vi "DC-DC_SC.vi"() -> ()   [LabVIEW 2025]
uses:
  controls/DC-DC-SC-2-enum.ctl
  controls/DC-DC-SC-2-cluster.ctl
  <vilib>/Utility/file.llb/Write Delimited Spreadsheet (string).vi
  <instrlib>/BK Precision 9200 Series/BK Precision 9200 Series.lvlib
panel:
  out "Time":u32
  in  "Current :":dbl
  in  "Voltage :":dbl
  in  "START":bool
  in  "BK_COM :":refnum<visa-resource-name>
  out "error out":errorcluster
  in  "error in (no error)":errorcluster
  in  "DATA":i32(listbox)
  in  "Exit":bool
  in  "Connect":bool
  # "DC-DC-Shorts"
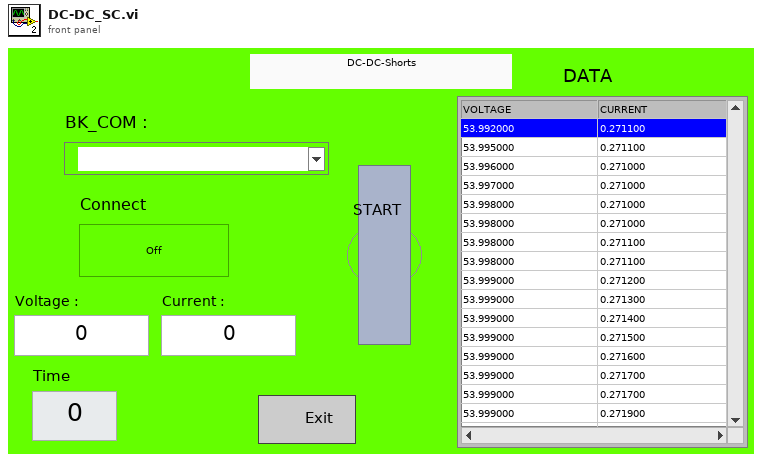
[diagram p1: front panel]
types:
  T1 = typedef "DC-DC-SC-2-cluster.ctl" = cluster{"File":path, "BK COM":refnum<visa-resource-name>, "Data":string[], "Stop":bool, "Start":bool, "Parameters":dbl[], "Seconds":u32}
  T2 = typedef "DC-DC-SC-2-enum.ctl" = enum16{"Init", "Poll", "Connect", "Set", "Start", "Read", "Stop", "Log", "Error", "Exit"}
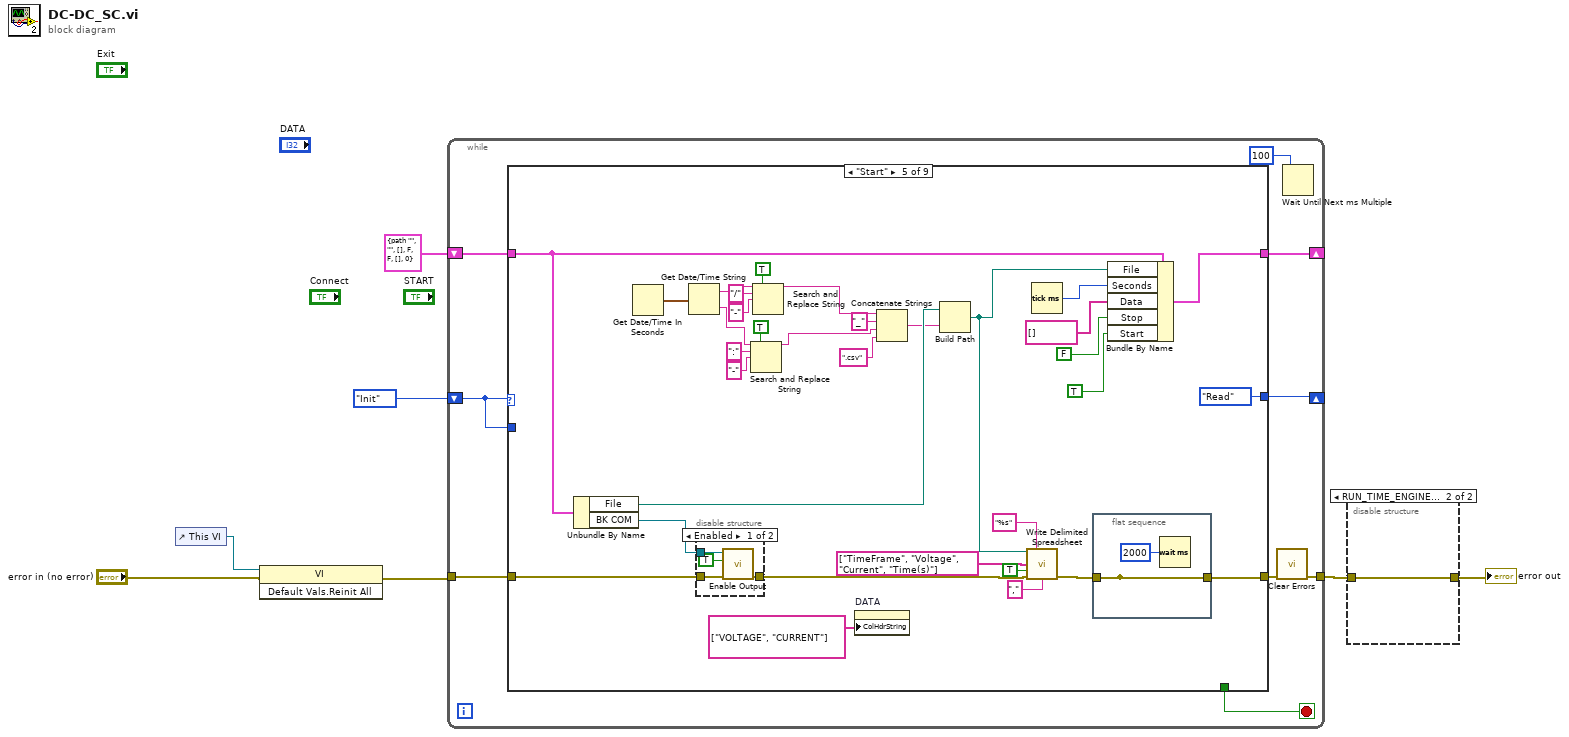
[diagram p0: block diagram]
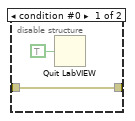
[diagram p2: hidden frame]
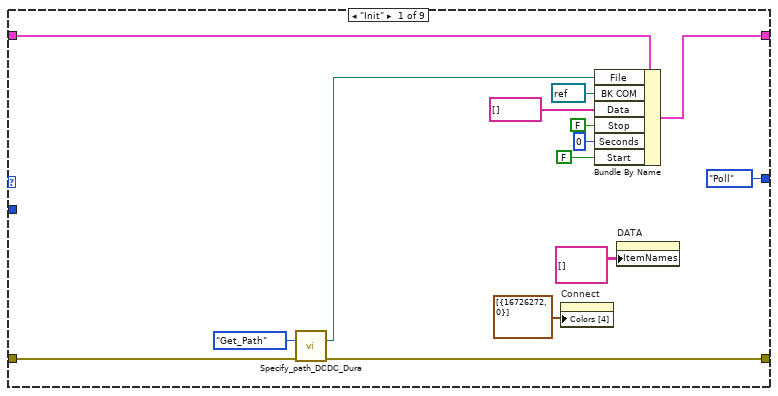
[diagram p3: hidden frame]
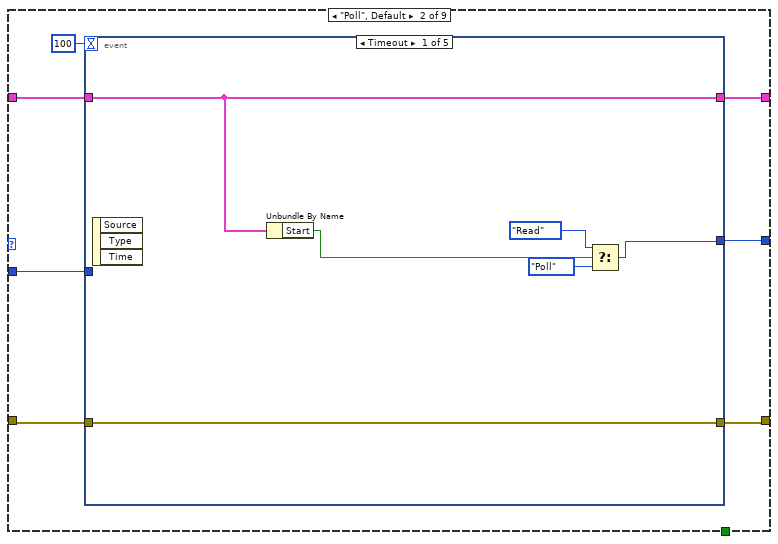
[diagram p4: hidden frame]
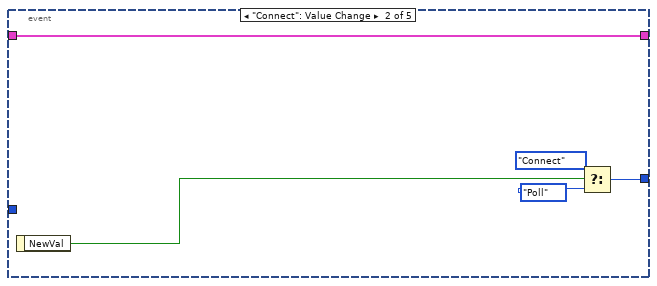
[diagram p5: hidden frame]
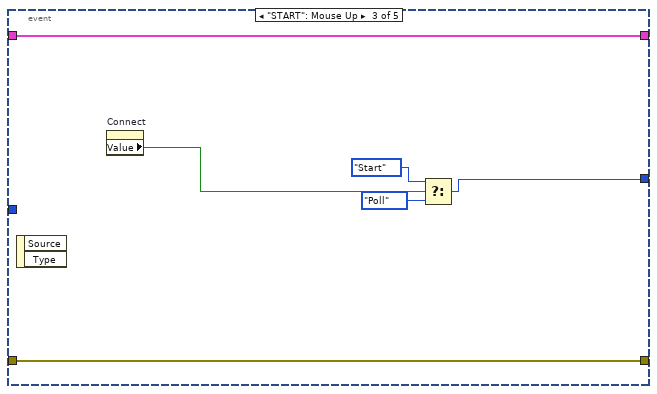
[diagram p6: hidden frame]
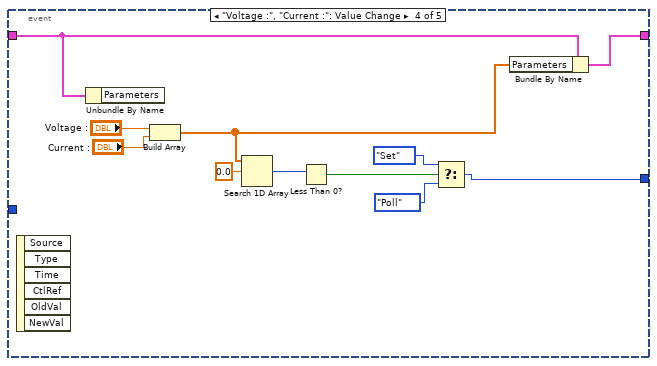
[diagram p7: hidden frame]
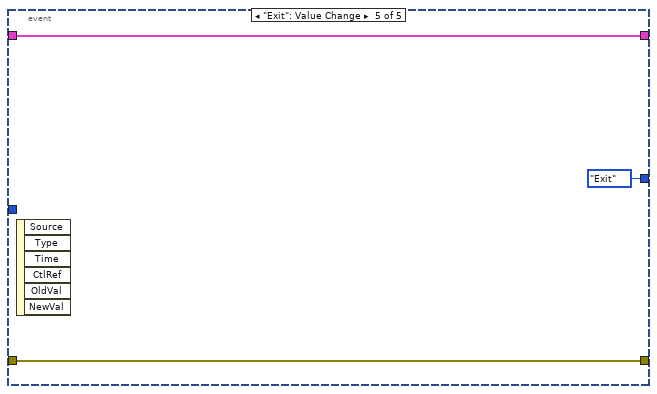
[diagram p8: hidden frame]
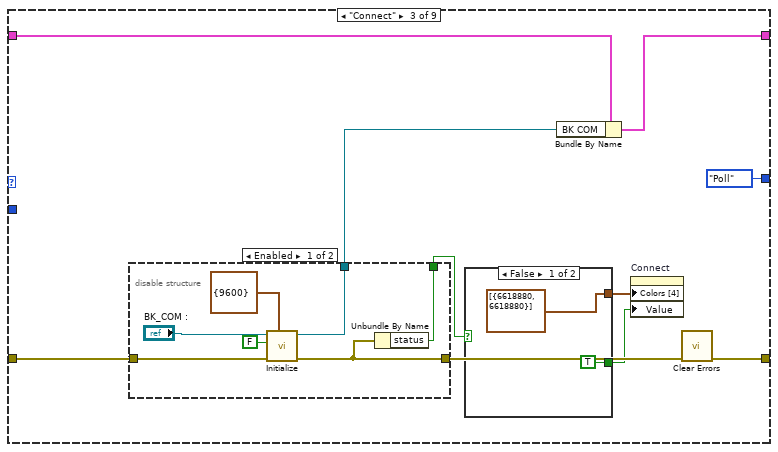
[diagram p9: hidden frame]
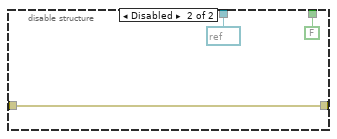
[diagram p10: hidden frame]
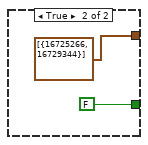
[diagram p11: hidden frame]
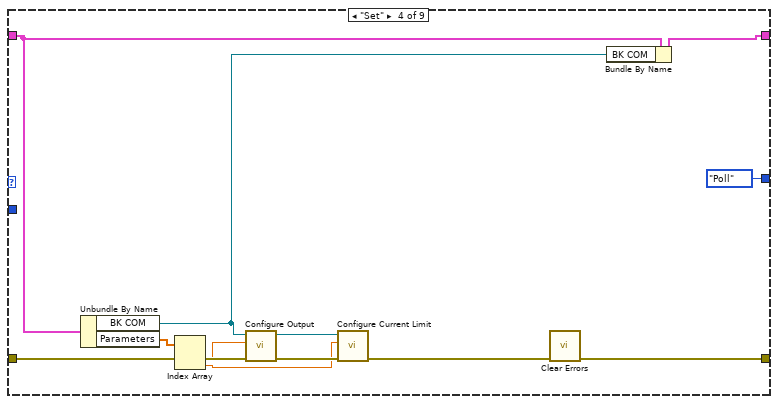
[diagram p12: hidden frame]
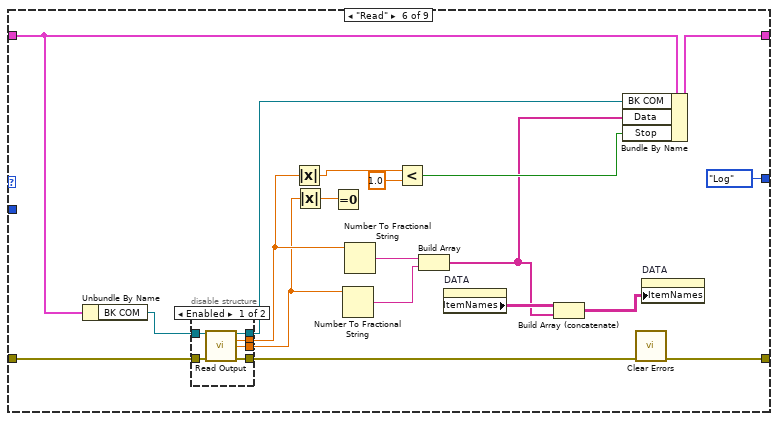
[diagram p14: hidden frame]
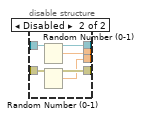
[diagram p15: hidden frame]
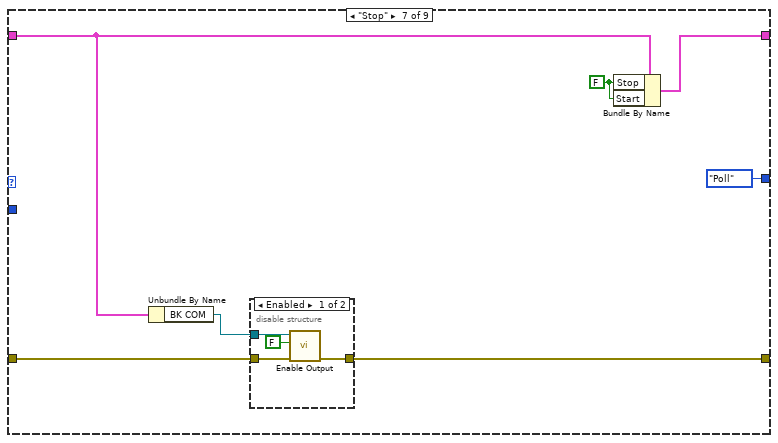
[diagram p16: hidden frame]
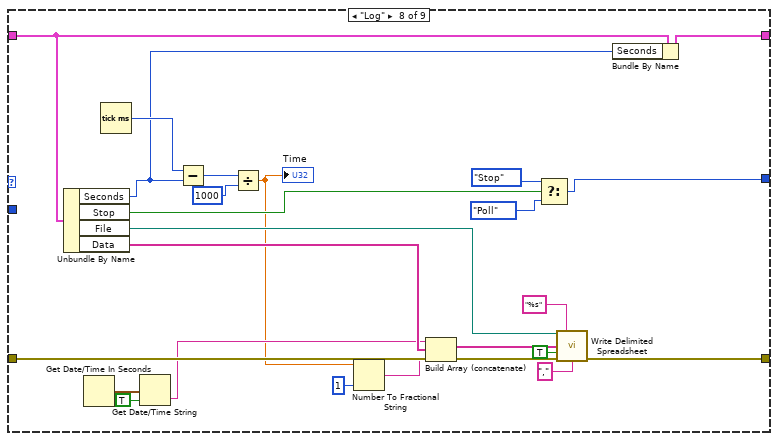
[diagram p18: hidden frame]
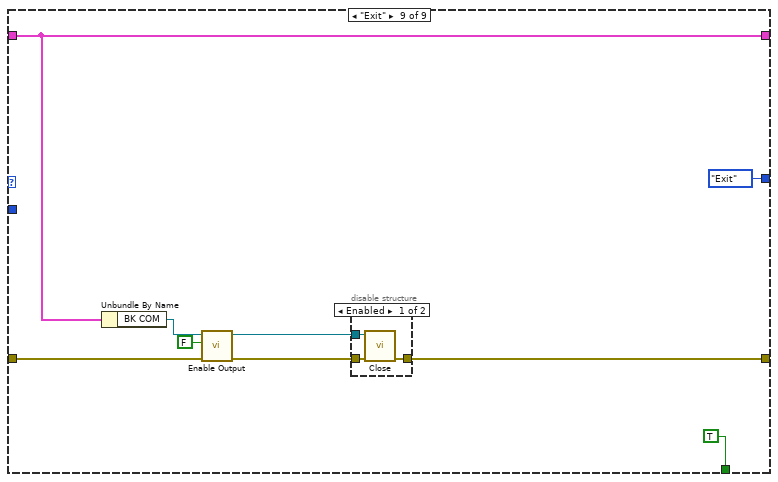
[diagram p19: hidden frame]
diagram:
  n1 = control-ref of="This VI"() -> (w5:refnum<vi>)
  n2 = invoke class="VI" method="Default Vals.Reinit All"(reference=w5, error in="error in (no error)") -> (error out=w3:errorcluster)  [unwired: 1 in, 2 out]
  n3 = while {
    shift-right: [w14] -> _
    shift-left: DC-DC-SC-2-enum."Init" -> [w8]
    shift-right: [w15] -> _
    shift-left: T1 {"File"=path "", "BK COM"="", "Data"=[], "Stop"=FALSE, "Start"=FALSE, "Parameters"=[], "Seconds"=0} -> [w16]
    tunnel: w3 -> [w12]
    tunnel: [w10] -> w2
    stop <- w13 stop-if-true
    n4 = case shown="\"Start\"" w8 {
      tunnel: w16 -> [w29 w36 w76 w96 w136 w162 w176 w198 w214]
      tunnel: [w28 w35 w75 w94 w133 w158 w179 w193 w214] -> w15
      tunnel: [DC-DC-SC-2-enum."Poll" ("f") w34 DC-DC-SC-2-enum."Poll" ("f") DC-DC-SC-2-enum."Poll" ("f") DC-DC-SC-2-enum."Read" ("f") DC-DC-SC-2-enum."Log" ("f") DC-DC-SC-2-enum."Poll" ("f") w199 DC-DC-SC-2-enum."Exit" ("f")] -> w14
      tunnel: [_ _ _ _ _ _ _ _ TRUE] -> w13
      tunnel: w12 -> [w27 w32 w78 w104 w137 w163 w178 w209 w216]
      tunnel: [w26 w33 w73 w97 w105 w159 w177 w208 w215] -> w11
      tunnel: w8 -> [_ w31 _ _ _ _ _ _ _]
      frame "Init" {
        n5 = call "Specify_path_DCDC_Dura.vi"("Path_Enum"=enum16{"Find_Path", "Get_Path"}."Get_Path", "error in (no error)"=w27) -> ("DATA"=w24:path, "error out"=w26:errorcluster)  [unwired: 7 in, 5 out]
        n6 = property on="Connect" class="Bool (strict)"("Colors [4]"=cluster{u32, u32}[] [{16726272, 0}]) -> ()  [unwired: 2 in, 2 out]
        n7 = Bundle By Name(cluster=w29, "File"=w24, "BK COM"=refnum<visa-resource-name> refnum, "Data"=string[] [], "Stop"=FALSE, "Seconds"=u32 0, "Start"=FALSE) -> (w28:T1)
        n8 = property on="DATA" class="MCListbox (strict)"("ItemNames"=string[][] [] ("Item Names")) -> ()  [unwired: 2 in, 2 out]
      }
      frame "Poll", Default {
        n9 = event shown="[0] Timeout" {
          selector: _ -> [_ _ _ _ _]
          dyn-events: _ -> [_ _ _ _ _]
          timeout: 100 -> [_ _ _ _ _]
          tunnel: w36 -> [w42 w48 w53 w61 w68]
          tunnel: [w42 w48 w53 w62 w68] -> w35
          tunnel: [w38 w45 w50 w63 DC-DC-SC-2-enum."Exit" ("f")] -> w34
          tunnel: [w43 _ w54 _ w66] -> w33
          tunnel: w32 -> [w43 _ w54 _ w66]
          tunnel: w31 -> [_ _ _ _ _]
          event Timeout {
            n10 = event-data() -> ()  [unwired: 1 in, 3 out]
            n11 = Unbundle By Name(w42) -> ("Start"=w41:bool)
            n12 = Select(t=DC-DC-SC-2-enum."Read", s=w41, f=DC-DC-SC-2-enum."Poll") -> (s? t:f=w38:T2)
          }
          event "Connect": Value Change {
            n13 = event-data() -> ("NewVal"=w47:bool)  [unwired: 1 in]
            n14 = Select(t=DC-DC-SC-2-enum."Connect", s=w47, f=DC-DC-SC-2-enum."Poll") -> (s? t:f=w45:T2)
          }
          event "START": Mouse Up {
            n15 = event-data() -> ()  [unwired: 1 in, 2 out]
            n16 = property on="Connect" class="Bool (strict)"() -> ("Value"=w52:bool)  [unwired: 2 in, 2 out]
            n17 = Select(t=DC-DC-SC-2-enum."Start" ("f"), s=w52, f=DC-DC-SC-2-enum."Poll") -> (s? t:f=w50:T2)
          }
          event "Voltage :", "Current :": Value Change {
            n18 = event-data() -> ()  [unwired: 1 in, 6 out]
            n19 = Unbundle By Name(w61) -> ()  [unwired: 1 out]
            n20 = Build Array("Voltage :", "Current :") -> (w55:dbl[])
            n21 = Search 1D Array(1D array=w55, element=0.0) -> (index of element=w57:i32)  [unwired: 1 in]
            n22 = Less Than 0?(x=w57) -> (x < 0?=w56:bool)
            n23 = Select(t=DC-DC-SC-2-enum."Set", s=w56, f=DC-DC-SC-2-enum."Poll") -> (s? t:f=w63:T2)
            n24 = Bundle By Name(cluster=w61, "Parameters"=w55) -> (w62:T1)
          }
          event "Exit": Value Change {
            n25 = event-data() -> ()  [unwired: 1 in, 6 out]
          }
        }
      }
      frame "Connect" {
        n26 = disable-structure shown="Enabled" {
          disable-tunnel: w78 -> [w85 w88]
          disable-tunnel: [w81 refnum<visa-resource-name> refnum ("VISA resource name out")] -> w74
          disable-tunnel: [w80 w88] -> w72
          disable-tunnel: [w79 FALSE ("status")] -> w71
          frame Enabled {
            n27 = call <instrlib>:"Initialize.vi"("Serial Configuration"=cluster{"Baud Rate":u32} {"Baud Rate"=9600}, "error in (no error)"=w85, "ID Query (True)"=FALSE, "VISA resource name"="BK_COM :") -> ("error out"=w80:errorcluster, "VISA resource name out"=w81:refnum<visa-resource-name>)  [unwired: 6 in]
            n28 = Unbundle By Name(w80) -> ("status"=w79:bool)
          }
          frame Disabled {
          }
        }
        n29 = case shown="False" w71 {
          tunnel: [cluster{u32, u32}[] [{6618880, 6618880}] ("Colors [4]") cluster{u32, u32}[] [{16725266, 16729344}] ("Colors [4]")] -> w70
          tunnel: [TRUE ("Connect") FALSE ("Connect")] -> w69
          frame False {
          }
          frame True {
          }
        }
        n30 = Bundle By Name(cluster=w76, "BK COM"=w74) -> (w75:T1)
        n31 = property on="Connect" class="Bool (strict)"("Colors [4]"=w70, "Value"=w69) -> ()  [unwired: 2 in, 2 out]
        n32 = call <vilib>:"Clear Errors.vi"("error in (no error)"=w72) -> ("error out"=w73:errorcluster)  [unwired: 5 in, 1 out]
      }
      frame "Set" {
        n33 = Unbundle By Name(w96) -> ("BK COM"=w93:refnum<visa-resource-name>, "Parameters"=w102:dbl[])
        n34 = Index Array(array=w102) -> (element #1=w101:dbl, element #2=w99:dbl)  [unwired: 2 in]
        n35 = call <instrlib>:"Configure Output.vi"("error in (no error)"=w104, "Voltage Level (0.0 V)"=w101, "VISA resource name"=w93) -> ("error out"=w103:errorcluster, "VISA resource name out"=w98:refnum<visa-resource-name>)  [unwired: 7 in]
        n36 = call <instrlib>:"Configure Current Limit.vi"("error in (no error)"=w103, "Current Limit (0.0 A)"=w99, "VISA resource name"=w98) -> ("error out"=w100:errorcluster)  [unwired: 7 in, 1 out]
        n37 = call <vilib>:"Clear Errors.vi"("error in (no error)"=w100) -> ("error out"=w97:errorcluster)  [unwired: 5 in, 1 out]
        n38 = Bundle By Name(cluster=w96, "BK COM"=w93) -> (w94:T1)
      }
      frame "Start" {
        n39 = Unbundle By Name(w136) -> ("File"=w131:path, "BK COM"=w135:refnum<visa-resource-name>)
        n40 = Get Date/Time In Seconds() -> (seconds since 1Jan1904=w134:timestamp)
        n41 = Get Date/Time String(seconds (now)=w134) -> (date string=w126:string, time string=w119:string)  [unwired: 2 in]
        n42 = disable-structure shown="Enabled" {
          disable-tunnel: w137 -> [w143 w144]
          disable-tunnel: w135 -> [w142 _]
          disable-tunnel: [w140 w144] -> w111
          frame Enabled {
            n43 = call <instrlib>:"Enable Output.vi"("error in (no error)"=w143, "Enable Output (F: False)"=TRUE, "VISA resource name"=w142) -> ("error out"=w140:errorcluster)  [unwired: 7 in, 1 out]
          }
          frame Disabled {
          }
        }
        n44 = Search and Replace String(replace all?=TRUE ("replace all? (F)"), input string=w119, search string=":", replace string="-" ("replace string (\"\")")) -> (result string=w116:string)  [unwired: 4 in, 3 out]
        n45 = Search and Replace String(replace all?=TRUE ("replace all? (F)"), input string=w126, search string="/", replace string="-" ("replace string (\"\")")) -> (result string=w118:string)  [unwired: 4 in, 3 out]
        n46 = property on="DATA" class="MCListbox (strict)"("ColHdrString"=string[] ["VOLTAGE", "CURRENT"] ("Column Header Strings[]")) -> ()  [unwired: 2 in, 2 out]
        n47 = Concatenate Strings(w118, "_" ("string"), w116, ".csv") -> (w127:string)
        n48 = Build Path(base path=w131, name or relative path=w127) -> (appended path=w110:path)
        n49 = call-poly <vilib>:"Write Delimited Spreadsheet.vi"("file path (dialog if empty)"=w110, "format (%s)"="%s" ("format (%.3f)"), "1D data"=string[] ["TimeFrame", "Voltage", "Current", "Time(s)"] ("Column Header Strings[]"), "append to file? (new file:F)"=TRUE, "error in (no error)"=w111, "delimiter (\\t)"="," ("delimiter (\\t)")) -> ("error out"=w106:errorcluster)  [unwired: 8 in, 1 out]
        n50 = Tick Count (ms)() -> (millisecond timer value=w132:u32)
        n51 = flat-sequence {
          tunnel: w106 -> [w139]
          tunnel: [w139] -> _
          tunnel: [w139] -> w105
          frame #0 {
            n52 = Wait (ms)(milliseconds to wait=u32 2000) -> ()  [unwired: 1 out]
          }
        }
        n53 = Bundle By Name(cluster=w136, "File"=w110, "Seconds"=w132, "Data"=string[] [], "Stop"=FALSE, "Start"=TRUE) -> (w133:T1)
      }
      frame "Read" {
        n54 = Unbundle By Name(w162) -> ("BK COM"=w161:refnum<visa-resource-name>)
        n55 = disable-structure shown="Enabled" {
          disable-tunnel: w163 -> [w169 w173]
          disable-tunnel: w161 -> [w168 w172]
          disable-tunnel: [w167 w173] -> w160
          disable-tunnel: [w166 w172] -> w155
          disable-tunnel: [w165 w171] -> w154
          disable-tunnel: [w164 w170] -> w151
          frame Enabled {
            n56 = call <instrlib>:"Read Output.vi"("VISA resource name"=w168, "error in (no error)"=w169) -> ("VISA resource name out"=w166:refnum<visa-resource-name>, "Actual Voltage Level (V)"=w165:dbl, "Actual Current Level (A)"=w164:dbl, "error out"=w167:errorcluster)  [unwired: 9 in, 1 out]
          }
          frame Disabled {
            n57 = Random Number (0-1)() -> (number: 0 to 1=w171:dbl)
            n58 = Random Number (0-1)() -> (number: 0 to 1=w170:dbl)
          }
        }
        n59 = Absolute Value(x=w154) -> (abs(x)=w146:dbl)
        n60 = Absolute Value(x=w151) -> (abs(x)=w152:dbl)
        n61 = Equal To 0?(x=w152) -> ()  [unwired: 1 out]
        n62 = Number To Fractional String(number=w151) -> (F-format string=w156:string)  [unwired: 3 in]
        n63 = Number To Fractional String(number=w154) -> (F-format string=w157:string)  [unwired: 3 in]
        n64 = Less?(x=w146, y=1.0) -> (x < y?=w153:bool)
        n65 = Build Array(w157, w156) -> (w148:string[])
        n66 = property on="DATA" class="MCListbox (strict)"() -> ("ItemNames"=w149:string[][])  [unwired: 2 in, 2 out]
        n67 = Build Array (concatenate)(w149, w148) -> (w147:string[][])
        n68 = Bundle By Name(cluster=w162, "BK COM"=w155, "Data"=w148, "Stop"=w153) -> (w158:T1)
        n69 = call <vilib>:"Clear Errors.vi"("error in (no error)"=w160) -> ("error out"=w159:errorcluster)  [unwired: 5 in, 1 out]
        n70 = property on="DATA" class="MCListbox (strict)"("ItemNames"=w147) -> ()  [unwired: 2 in, 2 out]
      }
      frame "Stop" {
        w174 = FALSE ("Stop")
        n71 = Unbundle By Name(w176) -> ("BK COM"=w175:refnum<visa-resource-name>)
        n72 = disable-structure shown="Enabled" {
          disable-tunnel: w178 -> [w184 w185]
          disable-tunnel: [w183 w185] -> w177
          disable-tunnel: w175 -> [w182 _]
          frame Enabled {
            n73 = call <instrlib>:"Enable Output.vi"("error in (no error)"=w184, "Enable Output (F: False)"=FALSE, "VISA resource name"=w182) -> ("error out"=w183:errorcluster)  [unwired: 7 in, 1 out]
          }
          frame Disabled {
          }
        }
        n74 = Bundle By Name(cluster=w176, "Stop"=w174, "Start"=w174) -> (w179:T1)
      }
      frame "Log" {
        n75 = Unbundle By Name(w198) -> ("Seconds"=w190:u32, "Stop"=w202:bool, "File"=w207:path, "Data"=w204:string[])
        n76 = Get Date/Time In Seconds() -> (seconds since 1Jan1904=w197:timestamp)
        n77 = Tick Count (ms)() -> (millisecond timer value=w192:u32)
        n78 = Get Date/Time String(seconds (now)=w197, want seconds? (F)=TRUE) -> (time string=w194:string)  [unwired: 1 in, 1 out]
        n79 = Subtract(x=w192, y=w190) -> (x-y=w191:u32)
        n80 = Divide(x=w191, y=u32 1000) -> (x/y=w188:dbl)
        "Time" <- w188
        n81 = Number To Fractional String(number=w188, precision (6)=i16 1) -> (F-format string=w186:string)  [unwired: 2 in]
        n82 = Build Array (concatenate)(w194, w204, w186) -> (w195:string[])
        n83 = Select(t=DC-DC-SC-2-enum."Stop", s=w202, f=DC-DC-SC-2-enum."Poll") -> (s? t:f=w199:T2)
        n84 = call-poly <vilib>:"Write Delimited Spreadsheet.vi"("file path (dialog if empty)"=w207, "format (%s)"="%s" ("format (%.3f)"), "1D data"=w195, "append to file? (new file:F)"=TRUE, "error in (no error)"=w209, "delimiter (\\t)"="," ("delimiter (\\t)")) -> ("error out"=w208:errorcluster)  [unwired: 8 in, 1 out]
        n85 = Bundle By Name(cluster=w198, "Seconds"=w190) -> (w193:T1)
      }
      frame "Exit" {
        n86 = Unbundle By Name(w214) -> ("BK COM"=w212:refnum<visa-resource-name>)
        n87 = call <instrlib>:"Enable Output.vi"("error in (no error)"=w216, "Enable Output (F: False)"=FALSE, "VISA resource name"=w212) -> ("error out"=w213:errorcluster, "VISA resource name out"=w211:refnum<visa-resource-name>)  [unwired: 7 in]
        n88 = disable-structure shown="Enabled" {
          disable-tunnel: w213 -> [w221 w222]
          disable-tunnel: [w220 w222] -> w215
          disable-tunnel: w211 -> [w219 _]
          frame Enabled {
            n89 = call <instrlib>:"Close.vi"("error in (no error)"=w221, "VISA resource name"=w219) -> ("error out"=w220:errorcluster)  [unwired: 9 in]
          }
          frame Disabled {
          }
        }
      }
    }
    n90 = call <vilib>:"Clear Errors.vi"("error in (no error)"=w11) -> ("error out"=w10:errorcluster)  [unwired: 5 in, 1 out]
    n91 = Wait Until Next ms Multiple(millisecond multiple=u32 100) -> ()  [unwired: 1 out]
  }
  n92 = disable-structure shown="RUN_TIME_ENGINE==False, Default" {
    disable-tunnel: w2 -> [w224 w225]
    disable-tunnel: [w224 w225] -> w1
    frame condition #0 {
      n93 = Quit LabVIEW(quit? (T)=TRUE) -> ()
    }
    frame condition #1 (active) {
    }
  }
  "error out" <- w1
